vi "Override Error.vi"(10 "Error":errorcluster, 11 "Base Actor in":refnum<class "Base Actor.lvclass">) -> (3 "Base Actor out":refnum<class "Base Actor.lvclass">)   [LabVIEW 2020, in "jettl.lvlib" / "Actor.lvlib" / "Base Actor.lvclass"]
uses:
  Base Actor.lvclass
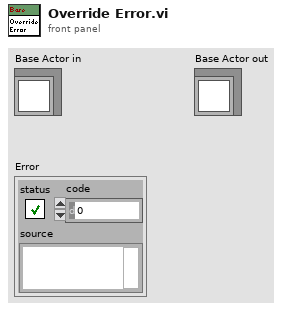
[diagram p1: front panel]
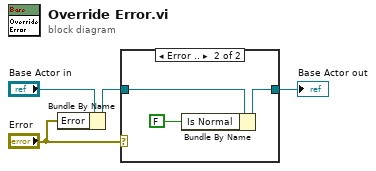
[diagram p0: block diagram]
diagram:
  n1 = Bundle By Name(cluster="Base Actor in", "Error"="Error") -> (w3:refnum<class "Base Actor.lvclass">)
  n2 = case shown="Error .." "Error" {
    tunnel: [w5 w7] -> w2
    tunnel: w3 -> [w5 w8]
    frame No Error {
    }
    frame Error {
      n3 = Bundle By Name(cluster=w8, "Is Normal"=FALSE) -> (w7:refnum<class "Base Actor.lvclass">)
    }
  }
  "Base Actor out" <- w2
